vi "Start Drag.vi"(0 "FSM.Label In":refnum<class "FSM.Label.lvclass">) -> (4 "FSM.Label Out":refnum<class "FSM.Label.lvclass">)   [LabVIEW 2020, in "FSM.Label.lvclass"]
uses:
  FSM.Label.lvclass
  FSM.Label.lvclass/FSM.Label.ctl
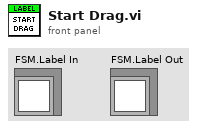
[diagram p1: front panel]
types:
  T1 = cluster{"left":i16, "top":i16, "right":i16, "bottom":i16}
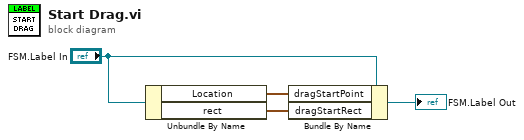
[diagram p0: block diagram]
diagram:
  n1 = Unbundle By Name("FSM.Label In") -> ("Location"=w3:cluster{"x":i16, "y":i16}, "rect"=w1:T1)
  n2 = Bundle By Name(cluster="FSM.Label In", "dragStartPoint"=w3, "dragStartRect"=w1) -> (→"FSM.Label Out":refnum<class "FSM.Label.lvclass">)
